vi "GananciasMotor2.vi"() -> ()   [LabVIEW 2024]
uses:
  <vilib>/Instr/_visa.llb/VISA Configure Serial Port (Instr).vi
  <vilib>/addons/control/pid/pid.llb/PID (DBL).vi
  <vilib>/addons/control/pid/NI_PID_pid.lvlib
panel:
  out "Waveform Chart":dynamicdata(graph)
  in  "PID G":cluster{"P":dbl, "I":dbl, "D":dbl}
  in  "Setpoint":dbl(slide) scale=0.0..100.0
  in  "stop":bool
  in  "baud rate (9600)":u32=9600
  in  "VISA resource name":refnum<visa-resource-name>
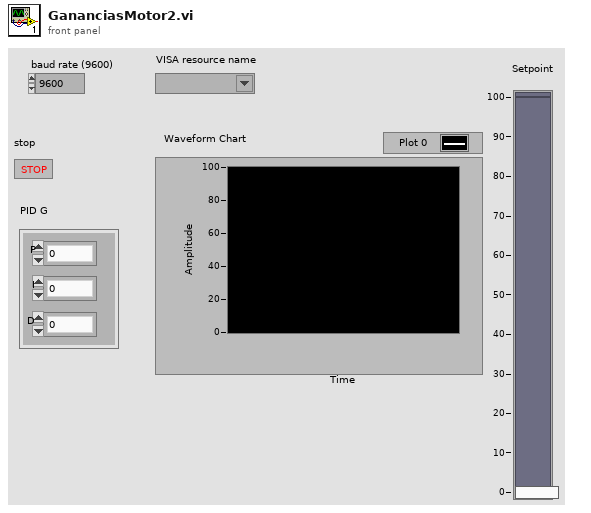
[diagram p1: front panel]
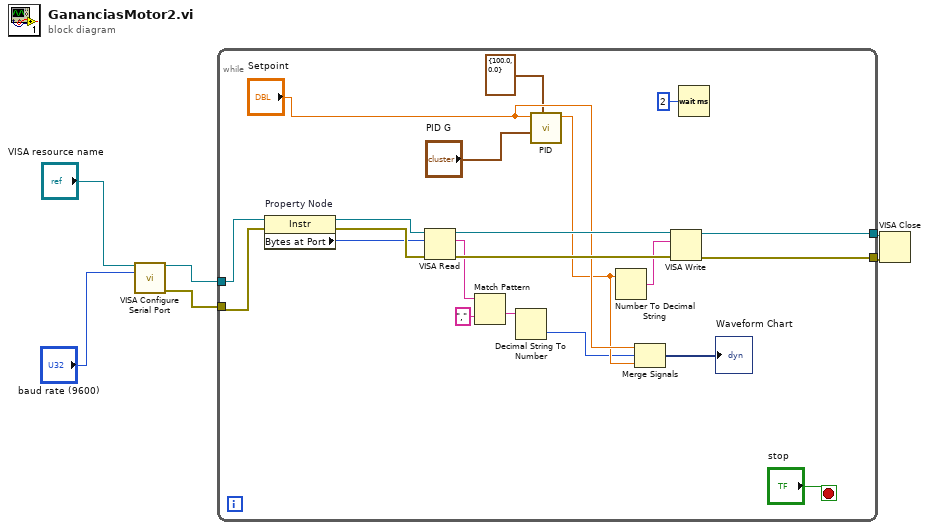
[diagram p0: block diagram]
diagram:
  n1 = call-poly "VISA Configure Serial Port"("VISA resource name"="VISA resource name", "baud rate (9600)"="baud rate (9600)") -> ("VISA resource name out"=w6:refnum<visa-resource-name>, "error out"=w5:errorcluster)  [unwired: 12 in]
  n2 = while {
    tunnel: w6 -> [w27]
    tunnel: w5 -> [w26]
    tunnel: [w24] -> w2
    tunnel: [w23] -> w1
    stop <- "stop" stop-if-true
    n3 = property on="Property Node" class="Instr"(reference=w27, error in=w26) -> (reference out=w21:refnum<visa-resource-name>, error out=w25:errorcluster, "Bytes at Port"=w19:u32)
    n4 = VISA Read(VISA resource name=w21, byte count=w19, error in (no error)=w25) -> (VISA resource name out=w16:refnum<visa-resource-name>, read buffer=w13:string, error out=w15:errorcluster)  [unwired: 1 out]
    n5 = Match Pattern(string=w13, regular expression=",") -> (after substring=w18:string)  [unwired: 1 in, 3 out]
    n6 = Decimal String To Number(string=w18) -> (number=w7:i32)  [unwired: 2 in, 1 out]
    n7 = call-poly <vilib>:"PID.vi"("output range"=cluster{"output high":dbl, "output low":dbl} {"output high"=100.0, "output low"=0.0}, "PID gains"="PID G", "setpoint"="Setpoint") -> ("output"=w8:dbl)  [unwired: 7 in, 1 out]
    n8 = Number To Decimal String(number=w8) -> (decimal integer string=w14:string)  [unwired: 1 in]
    n9 = Merge Signals("Setpoint", w7, w8) -> (→"Waveform Chart":dynamicdata)
    n10 = VISA Write(VISA resource name=w16, write buffer=w14, error in (no error)=w15) -> (VISA resource name out=w24:refnum<visa-resource-name>, error out=w23:errorcluster)  [unwired: 1 out]
    n11 = Wait (ms)(milliseconds to wait=u32 2) -> ()  [unwired: 1 out]
  }
  n12 = VISA Close(VISA resource name=w2, error in (no error)=w1) -> ()  [unwired: 1 out]
